vi "UIRef.vi"(8 "error in":errorcluster, 11 "group in":refnum<class "device.lvclass">) -> (0 "error out":errorcluster, 2 "VI refnum":refnum<vi>, 3 "group out":refnum<class "device.lvclass">)   [LabVIEW 2013, in "device.lvclass"]
uses:
  device.lvclass
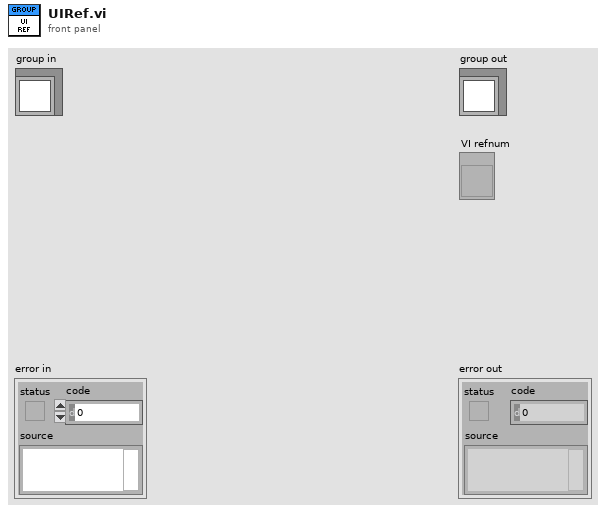
[diagram p1: front panel]
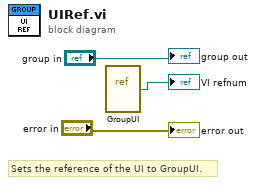
[diagram p0: block diagram]
diagram:
  # "Sets the reference of the UI to GroupUI."
  n1 = vi-ref "GroupUI.vi"() -> (→"VI refnum":refnum<vi>)
  "error out" <- "error in"
  "group out" <- "group in"
